vi "data_grid_v128.vi"(8 "No. Columns":i32=8, 9 "No. Rows":i32=16, 11 "Sensor Data":dbl[][](array[numeric])) -> (1 "Y (GRID)":dbl[][](array[numeric]), 2 "X (GRID)":dbl[][](array[numeric]), 3 "Z (GRID)":dbl[][](array[numeric]), 4 "Mag_GRID":dbl[][](array[numeric]))   [LabVIEW 2018]
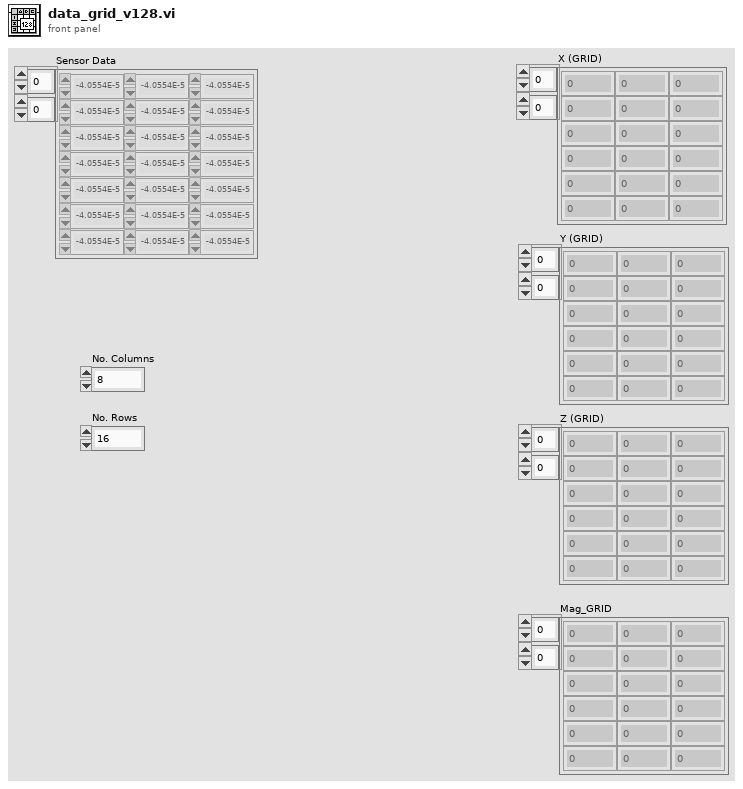
[diagram p1: front panel]
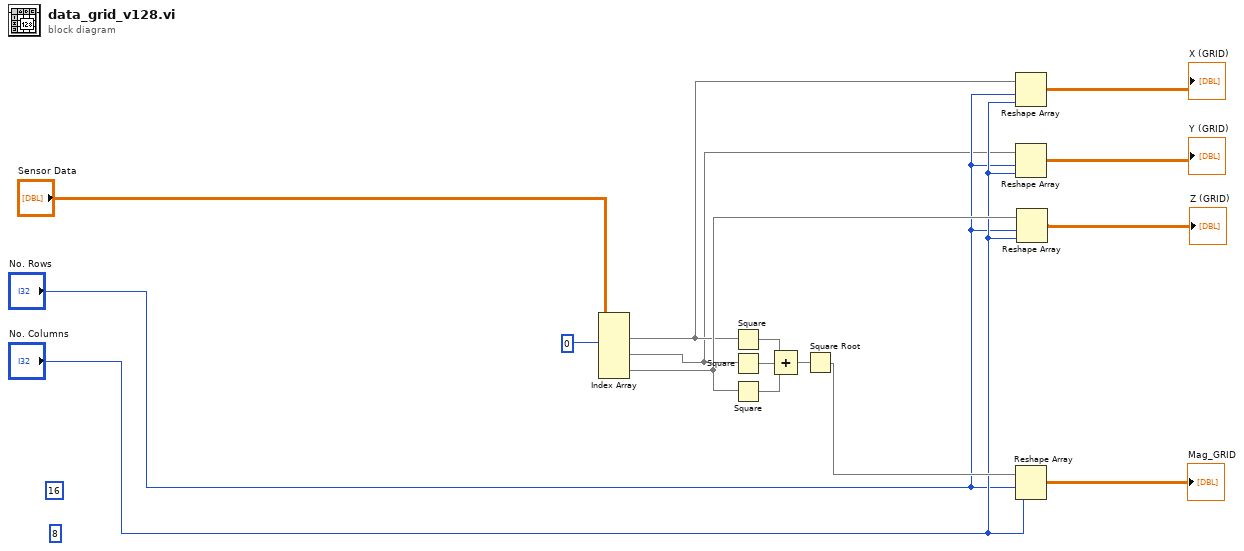
[diagram p0: block diagram]
diagram:
  (unwired) 16 ("dimension size")
  (unwired) 8 ("dimension size")
  n1 = Index Array(array="Sensor Data", index (col) #1=0 ("disabled index (col)")) -> (element #1=w4:dbl[], element #2=w3:dbl[], element #3=w8:dbl[])  [unwired: 5 in]
  n2 = Square(x=w4) -> (x^2=w15:dbl[])
  n3 = Square(x=w3) -> (x^2=w13:dbl[])
  n4 = Square(x=w8) -> (x^2=w14:dbl[])
  n5 = Compound Arithmetic op=ADD(w15, w13, w14) -> (w12:dbl[])
  n6 = Square Root(x=w12) -> (sqrt(x)=w11:dbl[])
  n7 = Reshape Array(w4, "No. Rows", "No. Columns") -> (→"X (GRID)":dbl[][])
  n8 = Reshape Array(w3, "No. Rows", "No. Columns") -> (→"Y (GRID)":dbl[][])
  n9 = Reshape Array(w11, "No. Rows", "No. Columns") -> (→"Mag_GRID":dbl[][])
  n10 = Reshape Array(w8, "No. Rows", "No. Columns") -> (→"Z (GRID)":dbl[][])
